vi "Upsample (CDB).vi"(9 "leading zeros":i32, 10 "upsampling factor":i32=1, 11 "X":cdb[](array[numeric])) -> (0 "error":i32, 3 "Upsampled Array":cdb[](array[numeric]))   [LabVIEW 2017, in "NI_AALPro.lvlib"]
doc: "Inserts zeros in input sequence <B>X</B> by <B>upsampling factor</B>. Wire data to the <B>X</B> input to determine the polymorphic instance to use or manually select the instance."
uses:
  NI_AALPro.lvlib
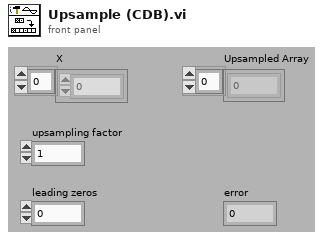
[diagram p1: front panel]
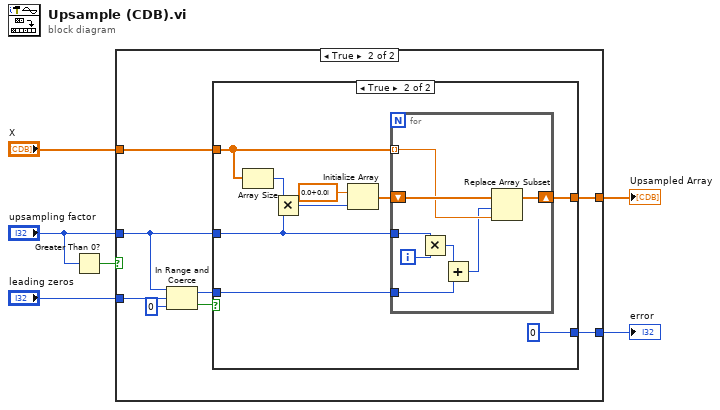
[diagram p0: block diagram]
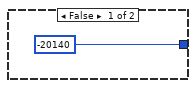
[diagram p2: hidden frame]
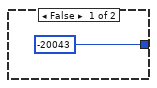
[diagram p3: hidden frame]
diagram:
  n1 = Greater Than 0?(x="upsampling factor") -> (x > 0?=w5:bool)
  n2 = case shown="True" w5 {
    tunnel: "X" -> [_ w15]
    tunnel: [_ w14] -> w6
    tunnel: "upsampling factor" -> [_ w13]
    tunnel: [-20140 ("error") w8] -> w3
    tunnel: "leading zeros" -> [_ w12]
    frame False {
    }
    frame True {
      n3 = In Range and Coerce(upper limit=w13, x=w12, lower limit=0) -> (coerced(x)=w9:i32, In Range?=w10:bool)
      n4 = case shown="True" w10 {
        tunnel: w15 -> [_ w18]
        tunnel: [_ w22] -> w14
        tunnel: w13 -> [_ w21]
        tunnel: w9 -> [_ w20]
        tunnel: [-20043 ("error") 0 ("error")] -> w8
        frame False {
        }
        frame True {
          n5 = Array Size(array=w18) -> (size(s)=w17:i32)
          n6 = Multiply(x=w17, y=w21) -> (x*y=w25:i32)
          n7 = Initialize Array(cdb 0.0+0.0i ("element"), w25) -> (w23:cdb[])
          n8 = for {
            shift-right: [w33] -> w22
            shift-left: w23 -> [w32]
            tunnel: w18 -> [w31] mode=indexing
            tunnel: w21 -> [w29]
            tunnel: w20 -> [w27]
            i -> [w30]
            n9 = Multiply(x=w29, y=w30) -> (x*y=w28:i32)
            n10 = Add(x=w28, y=w27) -> (x+y=w26:i32)
            n11 = Replace Array Subset(array=w32, new element=w31, index=w26) -> (w33:cdb[])
          }
        }
      }
    }
  }
  "Upsampled Array" <- w6
  "error" <- w3
